vi "Get Plugin Address.vi"(8 "error in (no error)":errorcluster, 11 "CIF_UI in":refnum<class "CIF_Manager_UI.lvclass">) -> (0 "error out":errorcluster, 2 "Plugin Address":string, 3 "CIF_UI out":refnum<class "CIF_Manager_UI.lvclass">)   [LabVIEW 2021, in "CIF_Manager_UI.lvclass"]
uses:
  CIF_Manager_UI.lvclass
  C:/Program Files/National Instruments/LabVIEW 2021/vi.lib/CIF Foundation/CIF Core/CIFUI/CIF_UI.lvclass
  CIF_Manager_UI.lvclass/CIF_Manager_UI.ctl
  <vilib>/CIF Foundation/CIF Core/CIFUI/CIF_UI.lvclass/CIF_UI.ctl
  <vilib>/CIF Foundation/CIF Core/CIFUI/Accessors/Read IP Address.vi
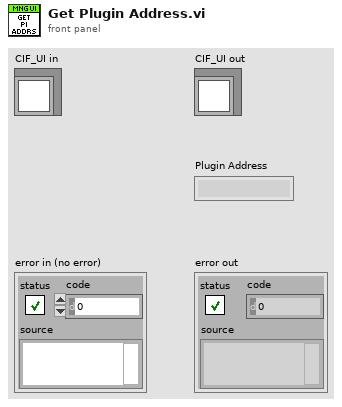
[diagram p1: front panel]
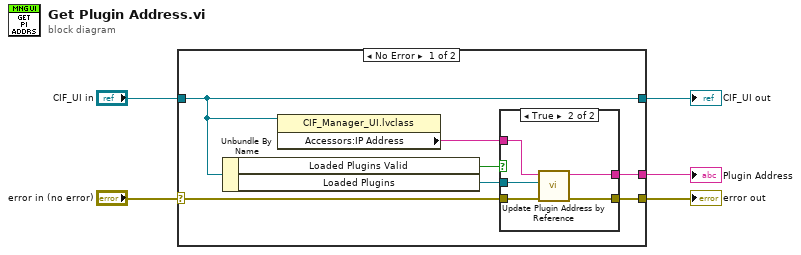
[diagram p0: block diagram]
diagram:
  n1 = case shown="No Error" "error in (no error)" {
    selector: "error in (no error)" -> [w9 w20]
    tunnel: [w11 w20] -> w4
    tunnel: [w7 w19] -> w2
    tunnel: "CIF_UI in" -> [w7 w19]
    tunnel: [w10 _] -> w1
    frame No Error {
      n2 = Unbundle By Name(w7) -> ("Loaded Plugins Valid"=w8:bool, "Loaded Plugins"=w12:refnum<vi>)
      n3 = property class="CIF_Manager_UI.lvclass"(reference=w7) -> ("Accessors:IP Address"=w6:string)  [unwired: 1 in, 2 out]
      n4 = case shown="True" w8 {
        tunnel: w12 -> [_ w18]
        tunnel: [w13 w17] -> w11
        tunnel: [_ w16] -> w10
        tunnel: w9 -> [w13 w15]
        tunnel: w6 -> [_ w14]
        frame False {
        }
        frame True {
          n5 = call "Update Plugin Address by Reference.vi"("error in (no error)"=w15, "Loaded Plugins"=w18, "IP"=w14) -> ("error out"=w17:errorcluster, "Plugin Address"=w16:string)  [unwired: 7 in]
        }
      }
    }
    frame Error {
    }
  }
  "error out" <- w4
  "CIF_UI out" <- w2
  "Plugin Address" <- w1
